vi "Empty Cluster.vi"() -> (0 "Empty Cluster":refnum<class "variant.lvclass">)   [LabVIEW 2020, in "JKI JSON Serialization.lvlib"]
uses:
  JKI JSON Serialization.lvlib
  OpenG-Variant-Data-Library/source/library/LVData/variant.lvclass
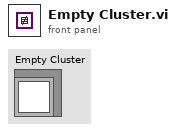
[diagram p1: front panel]
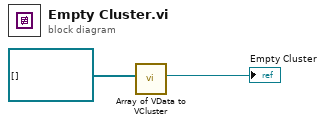
[diagram p0: block diagram]
diagram:
  n1 = call "Array of VData to VCluster.vi"("Array"=refnum<class "variant.lvclass">[] []) -> ("VCluster"=→"Empty Cluster":refnum<class "variant.lvclass">)  [unwired: 9 in, 1 out]
